vi "Get Session.vi"(8 "error in (no error)":errorcluster, 11 "FGen PXI Base CFG in":refnum<class "FGen PXI Base CFG.lvclass">) -> (0 "error out":errorcluster, 2 "Session":refnum<k15>, 3 "FGen PXI Base CFG out":refnum<class "FGen PXI Base CFG.lvclass">)   [LabVIEW 2023, in "FGen PXI Base CFG.lvlib" / "FGen PXI Base CFG.lvclass"]
uses:
  FGen PXI Base CFG.lvclass
  FGen PXI Base CFG.lvclass/FGen PXI Base CFG.ctl
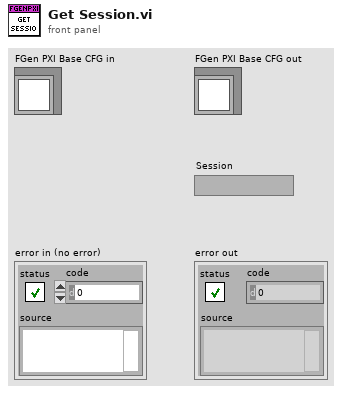
[diagram p1: front panel]
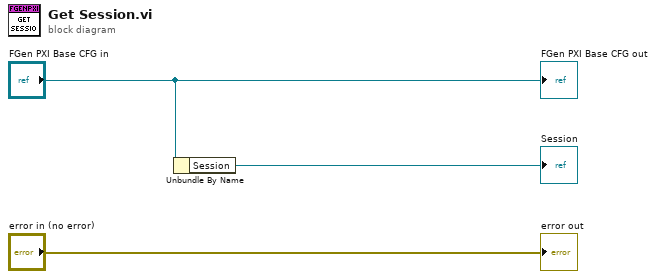
[diagram p0: block diagram]
diagram:
  n1 = Unbundle By Name("FGen PXI Base CFG in") -> ("Session"=→"Session":refnum<k15>)
  "error out" <- "error in (no error)"
  "FGen PXI Base CFG out" <- "FGen PXI Base CFG in"
